vi "build_paths.vi"(7 "Numeric":i32, 8 "name or relative path":string, 9 "path":path) -> (3 "appended path":path)   [LabVIEW 2018]
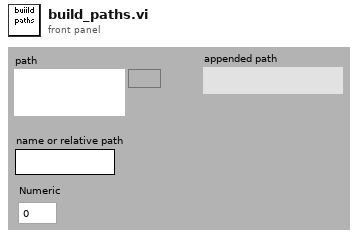
[diagram p1: front panel]
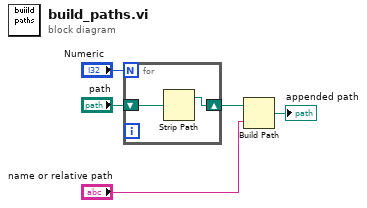
[diagram p0: block diagram]
diagram:
  n1 = for {
    N: "Numeric" -> [_]
    shift-right: [w6] -> w3
    shift-left: "path" -> [w7]
    n2 = Strip Path(path=w7) -> (stripped path=w6:path)  [unwired: 1 out]
  }
  n3 = Build Path(base path=w3, name or relative path="name or relative path") -> (appended path=→"appended path":path)
